vi "Écrire Operations.vi"(10 "Operations.lvclass":refnum<class "Operations.lvclass">, 11 "Portfolio en entrée":refnum<class "Portfolio.lvclass">) -> (3 "Portfolio en sortie":refnum<class "Portfolio.lvclass">)   [LabVIEW 2012, in "Portfolio.lvclass"]
uses:
  Portfolio.lvclass
  Operations/Operations.lvclass
  Portfolio.lvclass/Portfolio.ctl
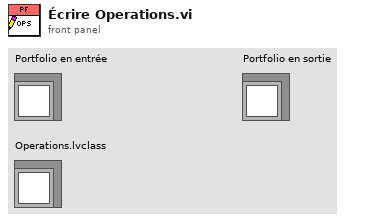
[diagram p1: front panel]
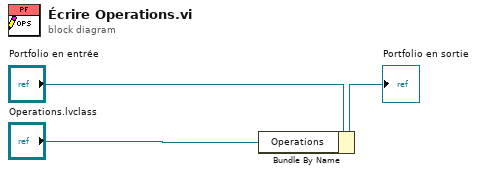
[diagram p0: block diagram]
diagram:
  n1 = Bundle By Name(cluster="Portfolio en entrée", "Operations"="Operations.lvclass") -> (→"Portfolio en sortie":refnum<class "Portfolio.lvclass">)
